vi "Pre Launch Init.vi"(11 "Client in":refnum<class "Client.lvclass">) -> (0 "error out":errorcluster, 3 "Client out":refnum<class "Client.lvclass">)   [LabVIEW 2021, in "Client.lvlib" / "Client.lvclass"]
doc: "(<B>Filename</B>: Actor Framework.lvlib:Actor.lvclass:Pre Launch Init.vi)\n\nDefines behavior that occurs after the Launch Nested Actor method is invoked but before the actor's Actor Core method begins running.\n\nBy default, this method does nothing. A descendant class may override it to define behavior."
uses:
  Client.lvclass
  Client.lvclass/Client.ctl
  <vilib>/ActorFramework/Actor/Actor.lvclass
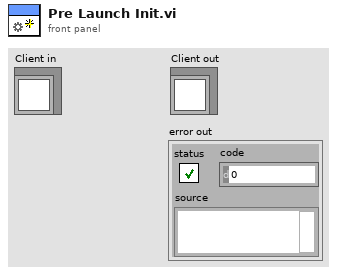
[diagram p1: front panel]
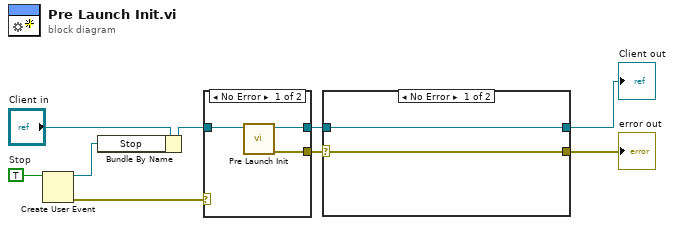
[diagram p0: block diagram]
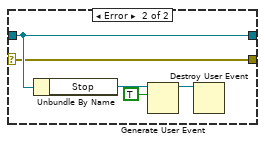
[diagram p2: hidden frame]
diagram:
  w8 = TRUE  # Stop
  n1 = Create User Event(user event datatype=w8) -> (user event=w6:refnum<user-event>, error out=w5:errorcluster)  [unwired: 1 in]
  n2 = Bundle By Name(cluster="Client in", "Stop"=w6) -> (w7:refnum<class "Client.lvclass">)
  n3 = case shown="No Error" w5 {
    selector: w5 -> [_ w13]
    tunnel: w7 -> [w12 w14]
    tunnel: [w11 w14] -> w4
    tunnel: [w10 w13] -> w3
    frame No Error {
      n4 = call-parent "Pre Launch Init.vi"("Actor in"=w12) -> ("error out"=w10:errorcluster, "Actor out"=w11:refnum<class "Client.lvclass">)  [unwired: 9 in]
    }
    frame Error {
    }
  }
  n5 = case shown="No Error" w3 {
    selector: w3 -> [w15 w17]
    tunnel: w4 -> [w16 w18]
    tunnel: [w16 w18] -> w2
    tunnel: [w15 w17] -> w1
    frame No Error {
    }
    frame Error {
      n6 = Unbundle By Name(w18) -> ("Stop"=w21:refnum<user-event>)
      n7 = Generate User Event(user event=w21, event data cluster=TRUE ("event data")) -> (user event out=w20:refnum<user-event>)  [unwired: 2 in, 1 out]
      n8 = Destroy User Event(user event=w20) -> ()  [unwired: 1 in, 1 out]
    }
  }
  "error out" <- w1
  "Client out" <- w2
